vi "0x52_Read_table_data.vi"(8 "error in":errorcluster, 9 "NTable":i32, 11 "paramUnicornIn":T1={"conParam"={"ReadIntParam"=TRUE, "ReadDescrParam"=FALSE, "ReadFloatParam"=TRUE, "debug"=FALSE, "ReadJSON"=TRUE, "IP_address"="192.168.1.216", "N_attempts"=3, "type_con"=enum."TCP", "MB_address"=1, "VISA"="COM1", "connection ID"=refnum, "nameDevices"="", "timeout"=3000, "port"=2000, "type_version"="0F0C0001", "baud_rate"=115200, "VersionControl"=TRUE, "TCP_conn"=TRUE, "WindowSize"=700}, "Param"={"NumParam"={"NTelem"=201, "NInt"=16, "NFloat"=10, "NTable"=2}, "ParamInt"=[{"ID"="Режим работы", "Num"=0, "Name"="", "Type"="", "Enum"="", "Desc"="", "Unit"="", "Access"="", "FormatStr"="", "Min"=0, "Max"=0}, {"ID"="", "Num"=0, "Name"="", "Type"="", "Enum"="", "Desc"="", "Unit"="", "Access"="", "FormatStr"="", "Min"=0, "Max"=0}, {"ID"="", "Num"=0, "Name"="", "Type"="", "Enum"="", "Desc"="", "Unit"="", "Access"="", "FormatStr"="", "Min"=0, "Max"=0}, {"ID"="", "Num"=0, "Name"="", "Type"="", "Enum"="", "Desc"="", "Unit"="", "Access"="", "FormatStr"="", "Min"=0, "Max"=0}, {"ID"="", "Num"=0, "Name"="", "Type"="", "Enum"="", "Desc"="", "Unit"="", "Access"="", "FormatStr"="", "Min"=0, "Max"=0}, {"ID"="", "Num"=0, "Name"="", "Type"="", "Enum"="", "Desc"="", "Unit"="", "Access"="", "FormatStr"="", "Min"=0, "Max"=0}, {"ID"="ModeWork", "Num"=0, "Name"="", "Type"="", "Enum"="", "Desc"="", "Unit"="", "Access"="", "FormatStr"="", "Min"=0, "Max"=0}], "Telemetry"=[], "Table"=[], "ParamFloat"=[]}}) -> (0 "error out":errorcluster, 2 "Array":sgl[][](array[numeric]), 3 "paramUnicornOut":T1={"conParam"={"ReadIntParam"=TRUE, "ReadDescrParam"=FALSE, "ReadFloatParam"=TRUE, "debug"=FALSE, "ReadJSON"=TRUE, "IP_address"="192.168.1.216", "N_attempts"=3, "type_con"=enum."TCP", "MB_address"=1, "VISA"="COM1", "connection ID"=refnum, "nameDevices"="", "timeout"=3000, "port"=2000, "type_version"="0F0C0001", "baud_rate"=115200, "VersionControl"=TRUE, "TCP_conn"=TRUE, "WindowSize"=700}, "Param"={"NumParam"={"NTelem"=201, "NInt"=16, "NFloat"=10, "NTable"=2}, "ParamInt"=[{"ID"="Режим работы", "Num"=0, "Name"="", "Type"="", "Enum"="", "Desc"="", "Unit"="", "Access"="", "FormatStr"="", "Min"=0, "Max"=0}, {"ID"="", "Num"=0, "Name"="", "Type"="", "Enum"="", "Desc"="", "Unit"="", "Access"="", "FormatStr"="", "Min"=0, "Max"=0}, {"ID"="", "Num"=0, "Name"="", "Type"="", "Enum"="", "Desc"="", "Unit"="", "Access"="", "FormatStr"="", "Min"=0, "Max"=0}, {"ID"="", "Num"=0, "Name"="", "Type"="", "Enum"="", "Desc"="", "Unit"="", "Access"="", "FormatStr"="", "Min"=0, "Max"=0}, {"ID"="", "Num"=0, "Name"="", "Type"="", "Enum"="", "Desc"="", "Unit"="", "Access"="", "FormatStr"="", "Min"=0, "Max"=0}, {"ID"="", "Num"=0, "Name"="", "Type"="", "Enum"="", "Desc"="", "Unit"="", "Access"="", "FormatStr"="", "Min"=0, "Max"=0}, {"ID"="ModeWork", "Num"=0, "Name"="", "Type"="", "Enum"="", "Desc"="", "Unit"="", "Access"="", "FormatStr"="", "Min"=0, "Max"=0}], "Telemetry"=[], "Table"=[], "ParamFloat"=[]}})   [LabVIEW 2017, in "LV_Unicorn.lvlib"]
uses:
  LV_Unicorn.lvlib
  Control/unicorn_Param.ctl
  Control/unicorn_conn.ctl
  Control/unicorn_JSON.ctl
  Control/unicorn_ParamInt.ctl
  Control/unicorn_Telemetry.ctl
  Control/unicorn_Table.ctl
  Control/unicorn_ParamFloat.ctl
panel:
  out "Чтение табличных данных":dbl(slide)=1.0 scale=0.0..100.0
  out "Номер табличного параметра":i32
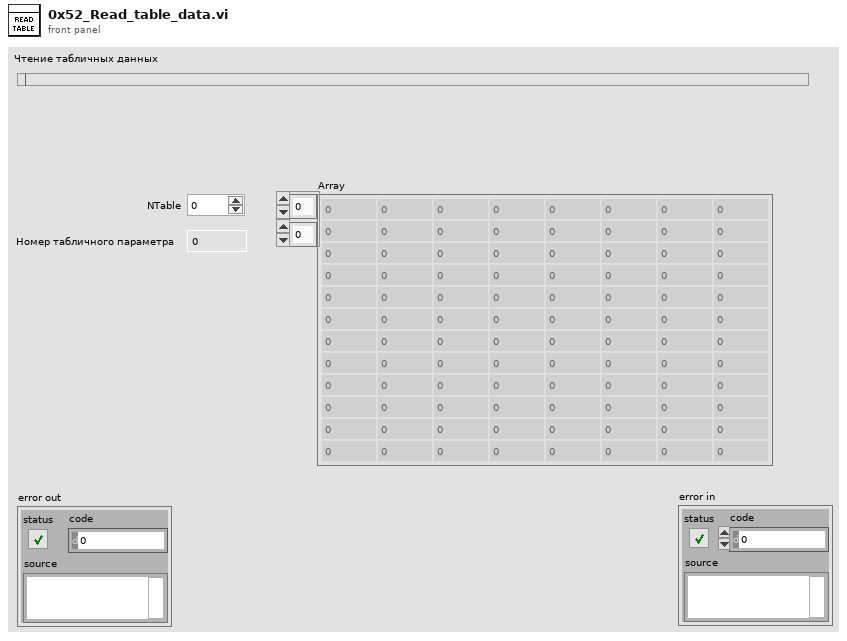
[diagram p1: front panel]
types:
  T1 = typedef "LV_Unicorn.lvlib/unicorn_Param.ctl" = cluster{"conParam":T2, "Param":T3}
  T2 = typedef "LV_Unicorn.lvlib/unicorn_conn.ctl" = cluster{"ReadIntParam":bool, "ReadDescrParam":bool, "ReadFloatParam":bool, "debug":bool, "ReadJSON":bool, "IP_address":string, "N_attempts":i32, "type_con":enum16{"Serial", "TCP"}, "MB_address":i32, "VISA":refnum<visa-resource-name>, "connection ID":refnum<k5>, "nameDevices":string, "timeout":i32, "port":u16, "type_version":string, "baud_rate":u32, "VersionControl":bool, "TCP_conn":bool, "WindowSize":i32}
  T3 = typedef "LV_Unicorn.lvlib/unicorn_JSON.ctl" = cluster{"NumParam":cluster{"NTelem":i32, "NInt":i32, "NFloat":i32, "NTable":i32}, "ParamInt":T4, "Telemetry":T5, "Table":T6, "ParamFloat":T7}
  T4 = typedef "LV_Unicorn.lvlib/unicorn_ParamInt.ctl" = cluster{"ID":string, "Num":i32, "Name":string, "Type":string, "Enum":string, "Desc":string, "Unit":string, "Access":string, "FormatStr":string, "Min":i32, "Max":i32}[]
  T5 = typedef "LV_Unicorn.lvlib/unicorn_Telemetry.ctl" = cluster{"ID":string, "Num":i32, "Name":string, "Desc":string, "Unit":string, "FormatStr":string, "Min":i32, "Max":i32}[]
  T6 = typedef "LV_Unicorn.lvlib/unicorn_Table.ctl" = cluster{"Num":i32, "Access":string, "ColumnCount":i32, "NeedParamPrepare":bool, "Columns":cluster{"Column":i32, "Desc":string, "Name":string}[], "DataType":string, "FormatStr":string, "ID":string, "Name":string, "RowCount":i32, "Rows":cluster{"Desc":string, "ID":string, "Max":i32, "Min":i32, "Name":string, "Row":i32, "Unit":string}[], "Type":string}[]
  T7 = typedef "LV_Unicorn.lvlib/unicorn_ParamFloat.ctl" = cluster{"ID":string, "Num":i32, "Name":string, "Type":string, "Enum":string, "Desc":string, "Unit":string, "Access":string, "FormatStr":string, "Min":sgl, "Max":sgl}[]
  T8 = cluster{"Режим":i32, "NumTable":i32, "Номер колонки":i32}
  T9 = cluster{"Num":i32, "Access":string, "ColumnCount":i32, "NeedParamPrepare":bool, "Columns":cluster{"Column":i32, "Desc":string, "Name":string}[], "DataType":string, "FormatStr":string, "ID":string, "Name":string, "RowCount":i32, "Rows":cluster{"Desc":string, "ID":string, "Max":i32, "Min":i32, "Name":string, "Row":i32, "Unit":string}[], "Type":string}
  T10 = cluster{"NumTable":i32, "Progress":i32, "TotalStep":i32, "RowCount":i32, "ColumCount":i32}
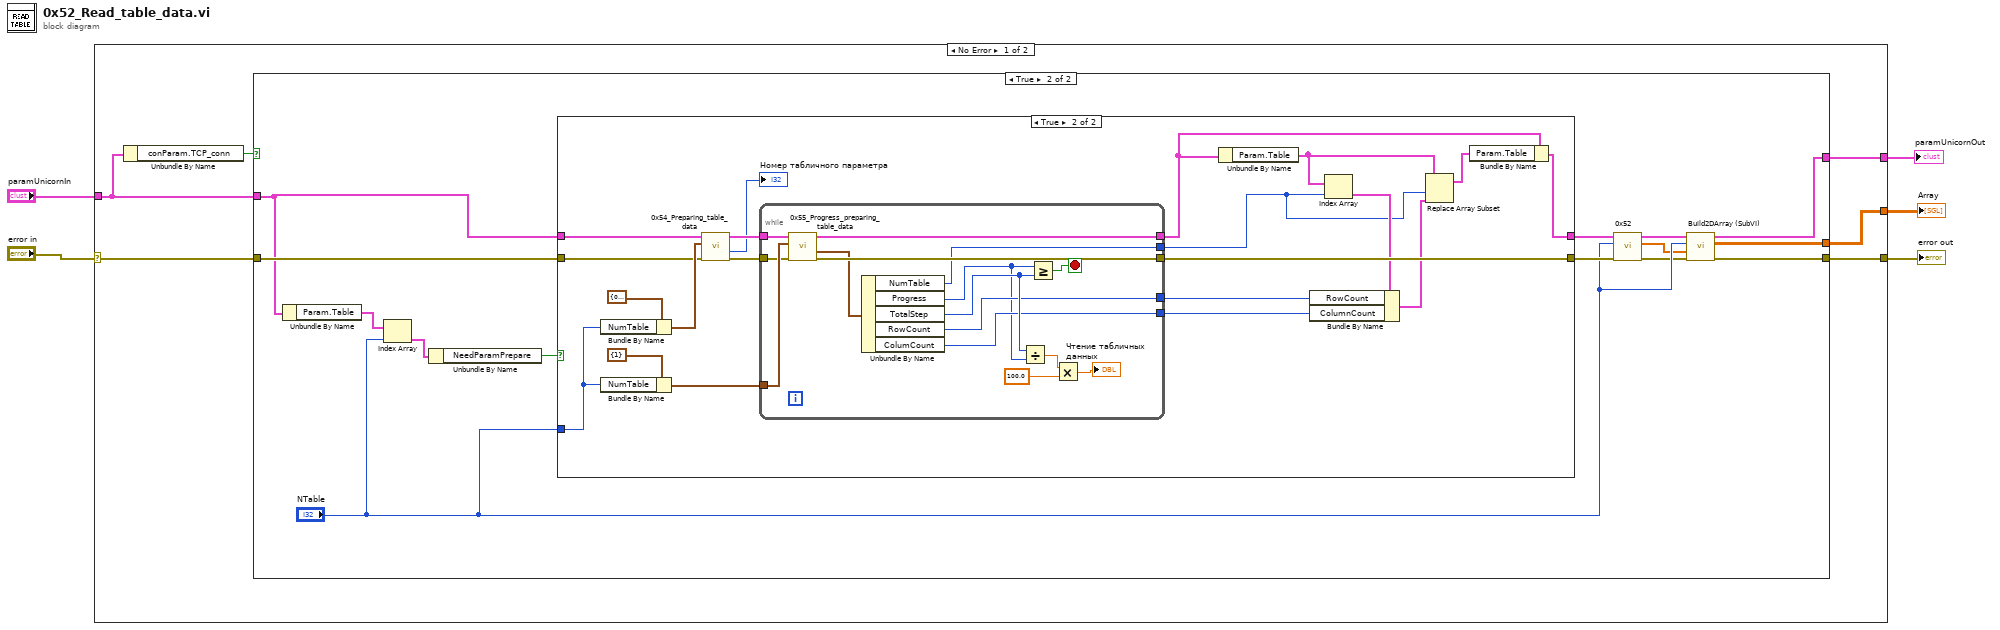
[diagram p0: block diagram]
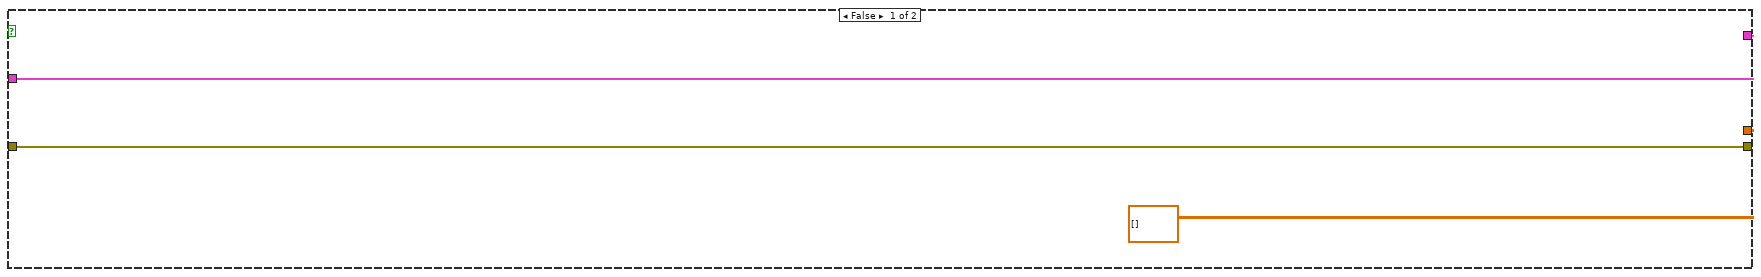
[diagram p2: hidden frame]
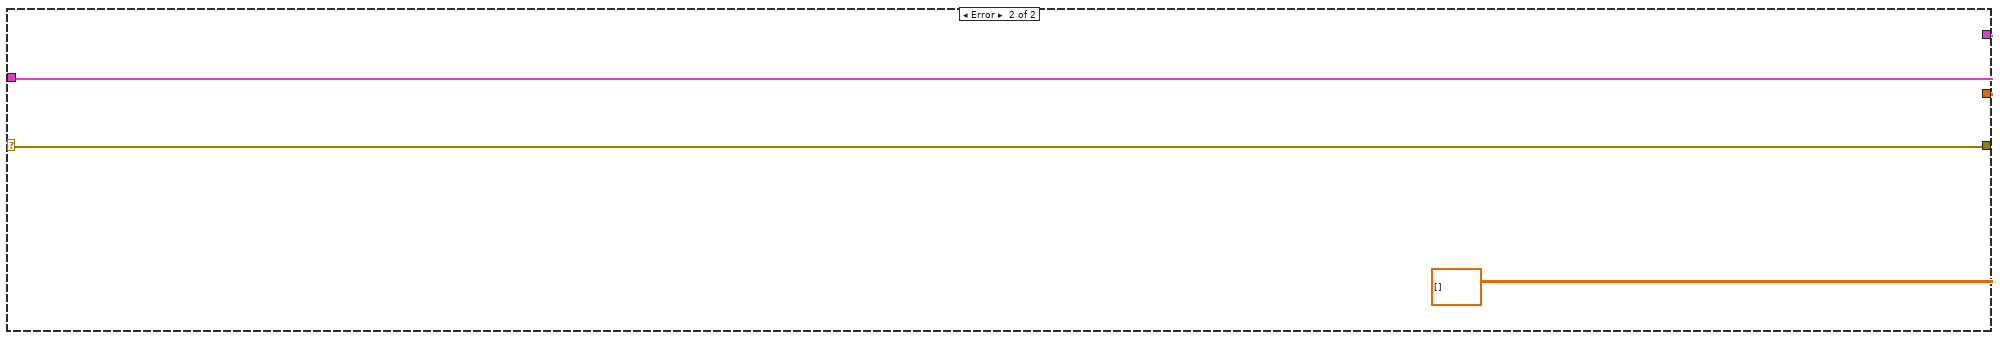
[diagram p4: hidden frame]
diagram:
  n1 = case shown="No Error" "error in" {
    selector: "error in" -> [w8 w67]
    tunnel: [w11 sgl[][] [] ("Array out")] -> w5
    tunnel: [w10 w67] -> w4
    tunnel: "paramUnicornIn" -> [w7 w68]
    tunnel: [w9 w68] -> w2
    frame No Error {
      n2 = Unbundle By Name(w7) -> ("conParam.TCP_conn"=w6:bool)
      n3 = case shown="True" w6 {
        tunnel: [sgl[][] [] ("Array out") w16] -> w11
        tunnel: [w13 w17] -> w10
        tunnel: w7 -> [w14 w15]
        tunnel: [w14 w18] -> w9
        tunnel: w8 -> [w13 w25]
        frame False {
        }
        frame True {
          n4 = Unbundle By Name(w15) -> ("Param.Table"=w28:T6)
          n5 = Index Array(array=w28, index="NTable") -> (element=w24:T9)
          n6 = Unbundle By Name(w24) -> ("NeedParamPrepare"=w23:bool)
          n7 = case shown="True" w23 {
            tunnel: "NTable" -> [_ w45]
            tunnel: [w29 w31] -> w22
            tunnel: w15 -> [w29 w44]
            tunnel: [w30 w43] -> w27
            tunnel: w25 -> [w30 w41]
            frame False {
            }
            frame True {
              n8 = Bundle By Name(cluster=T8 {"Режим"=0, "NumTable"=0, "Номер колонки"=-1} ("Param"), "NumTable"=w45) -> (w50:T8)
              n9 = Bundle By Name(cluster=cluster{"NumTable":i32} {"NumTable"=1} ("Param 3"), "NumTable"=w45) -> (w47:cluster{"NumTable":i32})
              n10 = call "0x54_Preparing_table_data.vi"("error in"=w41, "Param"=w50, "paramUnicorn"=w44) -> ("error out"=w42:errorcluster, "Номер табличного параметра"=→"Номер табличного параметра":i32, "paramUnicorn 2"=w46:T1)  [unwired: 4 in, 2 out]
              n11 = while {
                tunnel: w47 -> [w64]
                tunnel: [w54] -> w38
                tunnel: [w53] -> w37
                tunnel: w46 -> [w57]
                tunnel: [w65] -> w32
                tunnel: [w59] -> w43
                tunnel: w42 -> [w58]
                tunnel: [w51] -> w34
                stop <- w63 stop-if-true
                n12 = call "0x55_Progress_preparing_table_data.vi"("error in"=w58, "Param"=w64, "paramUnicorn 2"=w57) -> ("error out"=w59:errorcluster, "Cluster"=w56:T10, "paramUnicorn"=w65:T1)  [unwired: 4 in, 2 out]
                n13 = Unbundle By Name(w56) -> ("NumTable"=w51:i32, "Progress"=w52:i32, "TotalStep"=w55:i32, "RowCount"=w54:i32, "ColumCount"=w53:i32)
                n14 = Divide(x=w55, y=w52) -> (x/y=w62:dbl)
                n15 = Greater Or Equal?(x=w52, y=w55) -> (x >= y?=w63:bool)
                n16 = Multiply(x=w62, y=100.0) -> (x*y=→"Чтение табличных данных":dbl)
              }
              n17 = Unbundle By Name(w32) -> ("Param.Table"=w36:T6)
              n18 = Index Array(array=w36, index=w34) -> (element=w39:T9)
              n19 = Bundle By Name(cluster=w39, "RowCount"=w38, "ColumnCount"=w37) -> (w35:T9)
              n20 = Replace Array Subset(array=w36, new element=w35, index=w34) -> (w33:T6)
              n21 = Bundle By Name(cluster=w32, "Param.Table"=w33) -> (w31:T1)
            }
          }
          n22 = call "0x52.vi"("error in"=w27, "NTable"="NTable", "paramUnicorn"=w22) -> ("error out"=w20:errorcluster, "Table1D"=w19:sgl[], "paramUnicorn 2"=w21:T1)  [unwired: 5 in, 1 out]
          n23 = call "Build2DArray (SubVI).vi"("error in (no error)"=w20, "Array in"=w19, "Table"="NTable", "paramUnicornIn"=w21) -> ("error out"=w17:errorcluster, "Array out"=w16:sgl[][], "paramUnicornOut"=w18:T1)  [unwired: 5 in]
        }
      }
    }
    frame Error {
    }
  }
  "Array" <- w5
  "error out" <- w4
  "paramUnicornOut" <- w2
